vi "Realtime_interaction VI.vi"() -> ()   [LabVIEW 2020]
uses:
  <vilib>/FPGAPlugInAG/cRIO-9054/niLvFpga_Open_cRIO-9054.vi
  <vilib>/rvi/interface/common/dynamic/niFpgaDynamicAddResources.vi
  <vilib>/Utility/error.llb/Error Cluster From Error Code.vi
  <vilib>/rvi/errors/niLvFpgaAdjustHostInterfaceError.vi
  <vilib>/FPGAPlugInAG/Dynamic/niLvFpga_Close_Dynamic.vi
  <vilib>/rvi/interface/nirviOpenFPGA/nirviOpenFPGA.xnode
  FPGA Bitfiles/modifiedtestproj_FPGATarget_FPGAcontrolledVI_d33n4Chw7vI.lvbitx
  FPGA_controlled VI.vi
  <vilib>/rvi/interface/nirviReadWriteControl/nirviReadWriteControl.xnode
  <vilib>/rvi/interface/nirviCloseFPGA/nirviCloseFPGA.xnode
  NiFpgaLv.dll
  <vilib>/rvi/interface/Simulation/niFpgaSimulationCallBeginRW.vi
panel:
  out "Mod1/AI0":fxp<+/-,26,5>
  out "Numeric 2":fxp<+/-,20,5> format="%#_5f"
  in  "stop":bool
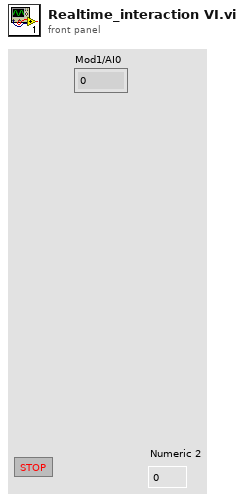
[diagram p1: front panel]
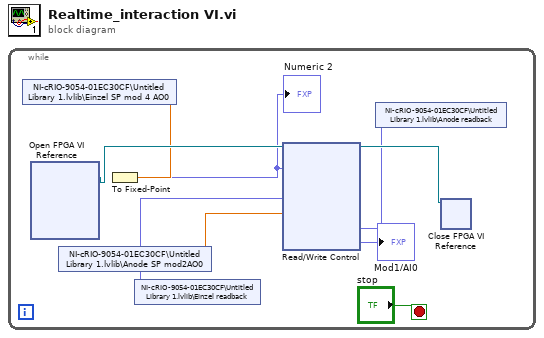
[diagram p0: block diagram]
diagram:
  n1 = while {
    stop <- "stop" stop-if-true
    n2 = shared-variable "NI-cRIO-9054-01EC30CF\\Untitled Library 1.lvlib\\Einzel SP mod 4 AO0"() -> (w4:dbl)  [unwired: 1 in, 1 out]
    n3 = xnode "Open FPGA VI Reference"() -> ("FPGA VI Reference Out"=w7:refnum<k20>)  [unwired: 2 in, 1 out]
    n4 = shared-variable "NI-cRIO-9054-01EC30CF\\Untitled Library 1.lvlib\\Anode SP mod2AO0"() -> (w2:dbl)  [unwired: 1 in, 1 out]
    n5 = To Fixed-Point(number=w4) -> (fixed-point=w3:fxp<+/-,20,5>)  [unwired: 1 in]
    "Numeric 2" <- w3
    n6 = xnode "Read/Write Control"("FPGA VI Reference In"=w7, "Mod4/AO0"=w3, "Mod2/AO0"=w2) -> ("FPGA VI Reference Out"=w5:refnum<k20>, "Mod1/AI0"=w6:fxp<+/-,26,5>, "Mod1/AI2"=w1:fxp<+/-,26,5>)  [unwired: 2 in, 2 out]
    "Mod1/AI0" <- w6
    n7 = shared-variable "NI-cRIO-9054-01EC30CF\\Untitled Library 1.lvlib\\Einzel readback"(w6) -> ()  [unwired: 1 in, 1 out]
    n8 = shared-variable "NI-cRIO-9054-01EC30CF\\Untitled Library 1.lvlib\\Anode readback"(w1) -> ()  [unwired: 1 in, 1 out]
    n9 = xnode "Close FPGA VI Reference"("FPGA VI Reference In"=w5) -> ()  [unwired: 1 in, 1 out]
  }
